vi "Pre Launch Init.vi"(11 "Screw in":refnum<class "Screw.lvclass">) -> (0 "error out":errorcluster, 3 "Screw out":refnum<class "Screw.lvclass">)   [LabVIEW 2018, in "Feeder Actor.lvlib" / "Screw.lvclass"]
doc: "(<B>Filename</B>: Actor Framework.lvlib:Actor.lvclass:Pre Launch Init.vi)\n\nDefines behavior that occurs after the Launch Nested Actor method is invoked but before the actor's Actor Core method begins running.\n\nBy default, this method does nothing. A descendant class may override it to define behavior."
uses:
  Screw.lvclass
  Screw.lvclass/Screw.ctl
  <vilib>/DAQmx/create/channels.llb/DAQmx Create Channel (CO-Pulse Generation-Frequency).vi
  <vilib>/DAQmx/configure/timing.llb/DAQmx Timing (Implicit).vi
  <vilib>/ActorFramework/Actor/Actor.lvclass
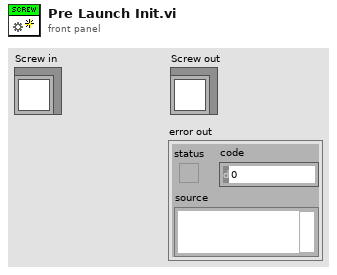
[diagram p1: front panel]
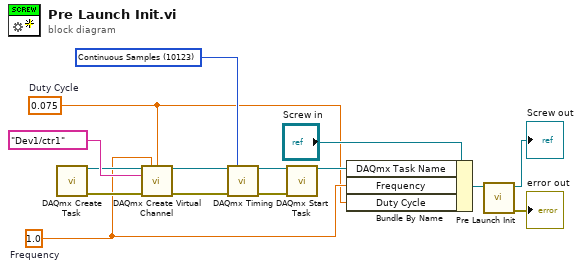
[diagram p0: block diagram]
diagram:
  w1 = 0.075  # Duty Cycle
  w6 = 10123 items=["Finite Samples"=10178, "Continuous Samples"=10123, "Hardware Timed Single Point"=12522] ("sample mode")
  w2 = 1.0  # Frequency
  n1 = call <vilib>:"DAQmx Create Task.vi"() -> ("task out"=w11:refnum<k21>, "error out"=w10:errorcluster)  [unwired: 14 in]
  n2 = call-poly <vilib>:"DAQmx Create Virtual Channel.vi"("task in"=w11, "frequency"=w2, "duty cycle"=w1, "counter"=tag "Dev1/ctr1" ("Counter(s) 2"), "error in"=w10) -> ("task out"=w13:refnum<k21>, "error out"=w8:errorcluster)  [unwired: 9 in]
  n3 = call-poly <vilib>:"DAQmx Timing.vi"("task/channels in"=w13, "sample mode"=w6, "error in"=w8) -> ("task out"=w9:refnum<k21>, "error out"=w7:errorcluster)  [unwired: 11 in]
  n4 = call <vilib>:"DAQmx Start Task.vi"("task/channels in"=w9, "error in"=w7) -> ("task out"=w3:refnum<k21>)  [unwired: 12 in, 1 out]
  n5 = Bundle By Name(cluster="Screw in", "DAQmx Task Name"=w3, "Frequency"=w2, "Duty Cycle"=w1) -> (w4:refnum<class "Screw.lvclass">)
  n6 = call-parent "Pre Launch Init.vi"("Actor in"=w4) -> ("error out"=→"error out":errorcluster, "Actor out"=→"Screw out":refnum<class "Screw.lvclass">)  [unwired: 9 in]
